vi "Linear Scaling.vi"(1 "Tag":T1 {"Vmax" min=-10.0 max=10.0 step=1.0; "Vmin" min=-10.0 max=10.0 step=1.0}, 2 "x":dbl) -> (0 "y":dbl)   [LabVIEW 2019]
panel:
  # "y=ax+b"
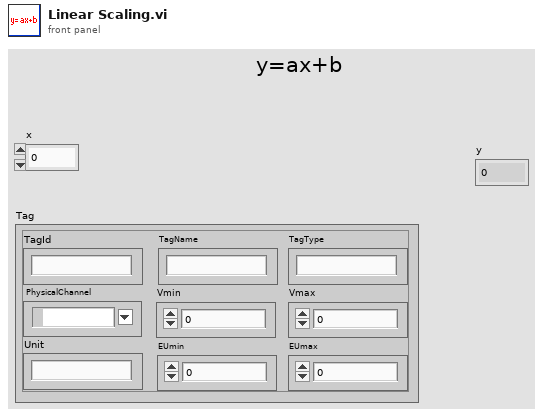
[diagram p1: front panel]
types:
  T1 = cluster{"TagId":string, "TagName":string, "TagType":string, "PhysicalChannel":tag, "Vmin":dbl, "Vmax":dbl, "Unit":string, "EUmin":dbl, "EUmax":dbl}
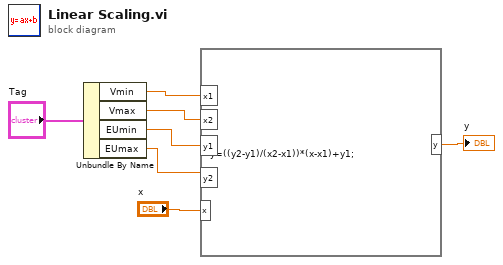
[diagram p0: block diagram]
diagram:
  n1 = Unbundle By Name("Tag") -> ("Vmin"=w4:dbl, "Vmax"=w3:dbl, "EUmin"=w2:dbl, "EUmax"=w1:dbl)
  n2 = formula code="y=((y2-y1)/(x2-x1))*(x-x1)+y1;"("x1"=w4, "y1"=w2, "x2"=w3, "y2"=w1, "x"="x") -> ("y"=→"y":dbl)
